vi "MessageName.vi"() -> (2 "MessageName":string)   [LabVIEW 2020, in "StartLog.lvlib"]
uses:
  StartLog.lvlib
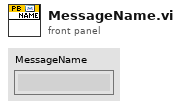
[diagram p1: front panel]
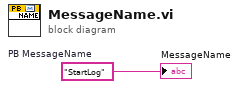
[diagram p0: block diagram]
diagram:
  w1 = "StartLog"  # PB MessageName
  "MessageName" <- w1
